vi "Final_DAQ_v2.vi"() -> ()   [LabVIEW 2019]
uses:
  src/class/mqtt/mqttTypedef/mqttBroker.ctl
  src/class/mqtt/mqttTypedef/mqttConnectionFlags.ctl
  src/class/mqtt/mqttTypedef/mqttWillInformation.ctl
  src/class/mqtt/mqttConfigFunction.ctl
  src/class/mqtt/mqttTXqueue/mqttTXdataQueueFunction.ctl
  src/class/mqtt/mqttTXqueue/mqttRXsubscriptionEventFunction.ctl
  src/class/mqtt/mqtt.lvclass
panel:
  out "電暖爐":bool
  out "電扇":bool
  out "電燈":bool
  out "開門 Flag":bool
  out "電暖爐-M":bool
  out "電扇-M":bool
  out "開門":bool
  out "電燈-M":bool
  out "溫度過低":bool
  out "溫度過高":bool
  out "Boolean":bool
  out "old-temp":dbl
  out "Numeric 2":dbl
  out "subscripts-status":bool
  out "Publish Topic":string
  out "Publish Data":string
  out "溫度上限(*C)":dbl
  out "溫度下限(*C)":dbl
  out "Subscripts Topic":string
  out "Subscripts Data":string
  out "F-format string":string
  out "now-temp":dbl
  out "Thermometer":dbl(slide) scale=0.0..40.0
  in  "stop":bool
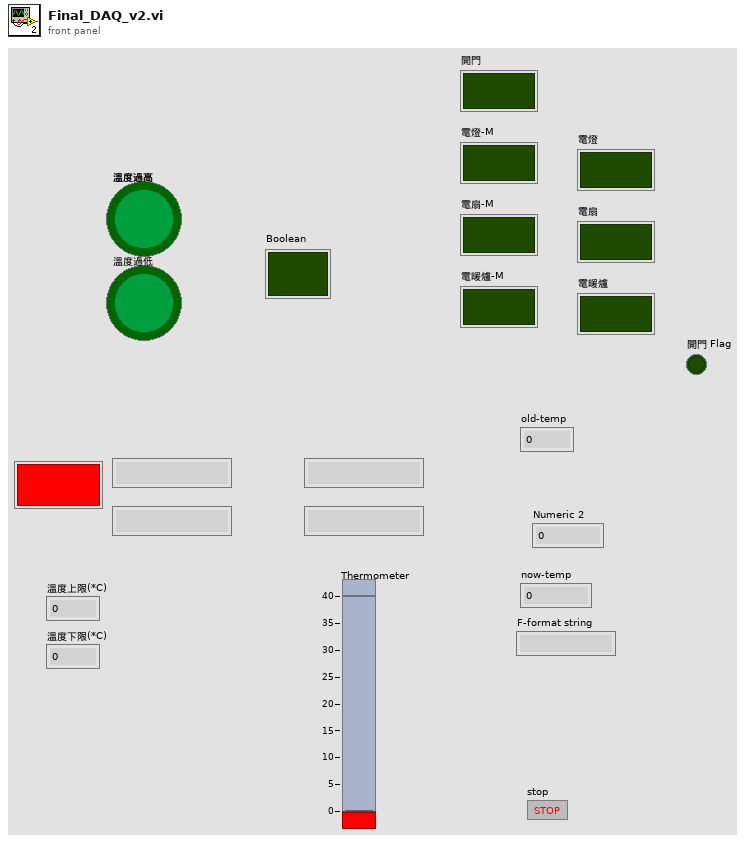
[diagram p1: front panel]
types:
  T1 = typedef "mqttRXsubscriptionEventFunction.ctl" = enum16{"init", "deinit", "getEventRef", "event"}
  T2 = typedef "mqttTXdataQueueFunction.ctl" = enum16{"init", "deinit", "getQueue", "enqueue"}
  T3 = typedef "mqtt.lvclass/mqttConfigFunction.ctl" = enum16{"init", "deinit", "set", "get"}
  T4 = typedef "mqttWillInformation.ctl" = cluster{"User Name":string, "Password":string}
  T5 = typedef "mqttConnectionFlags.ctl" = cluster{"reserved":bool, "clean session":bool, "will flag":bool, "willQOS":enum8{"At most once", "At least once", "Exactly once", "Reserved"}, "will retain":bool, "password":bool, "user name":bool}
  T6 = typedef "mqttBroker.ctl" = cluster{"address":string, "port":u16, "connTimeout":i32, "writeTimeout":i32, "readTimeout":i32, "subTimeout":i32}
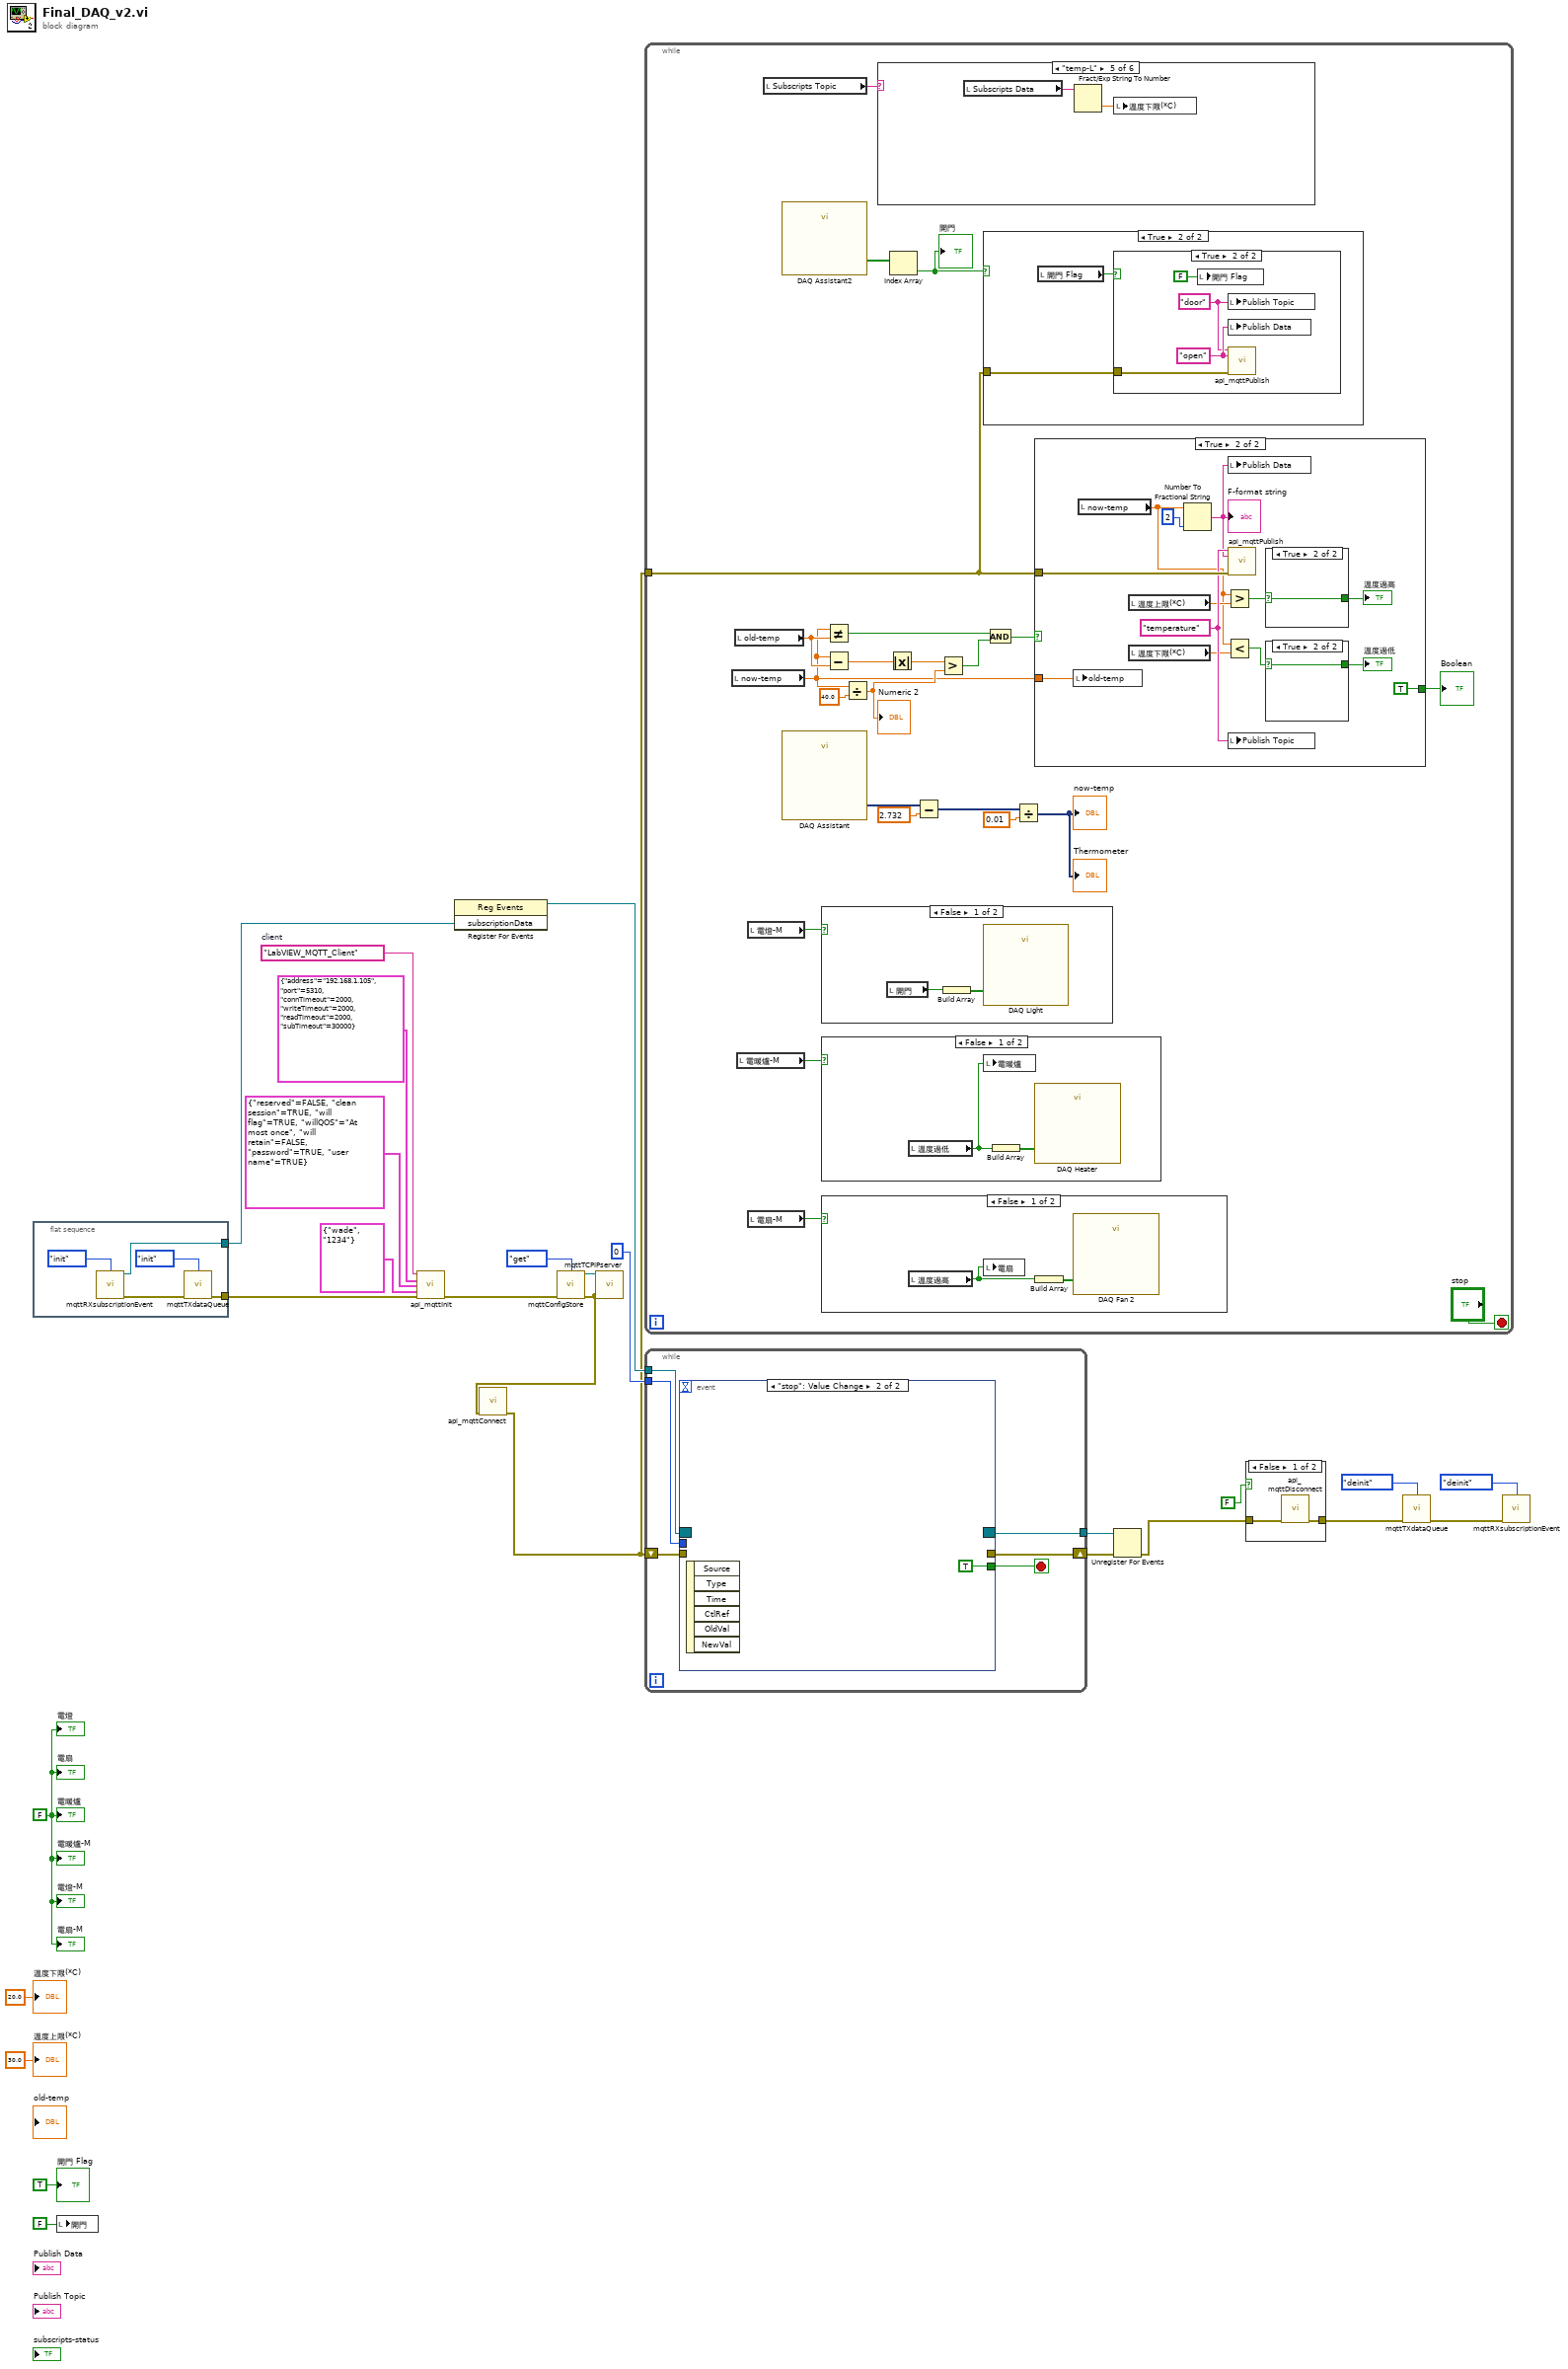
[diagram p0: block diagram]
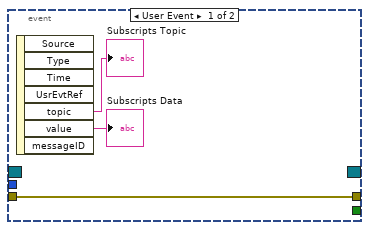
[diagram p3: hidden frame]
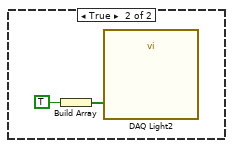
[diagram p4: hidden frame]
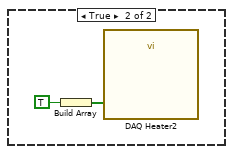
[diagram p5: hidden frame]
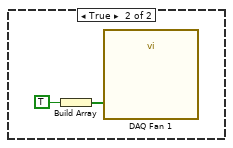
[diagram p6: hidden frame]
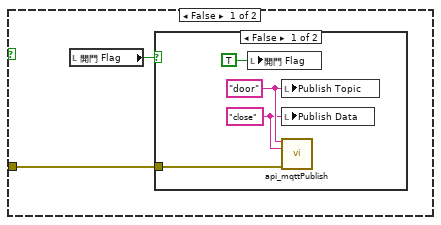
[diagram p7: hidden frame]
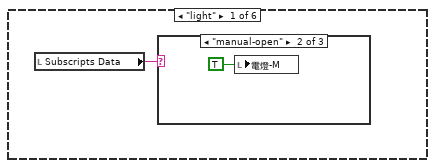
[diagram p10: hidden frame]
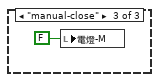
[diagram p12: hidden frame]
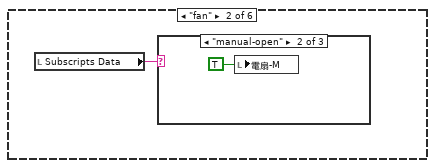
[diagram p13: hidden frame]
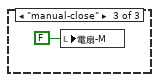
[diagram p15: hidden frame]
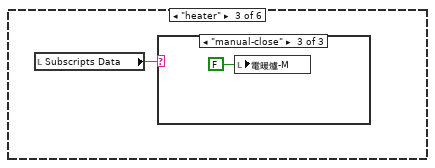
[diagram p16: hidden frame]
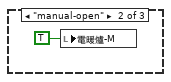
[diagram p18: hidden frame]
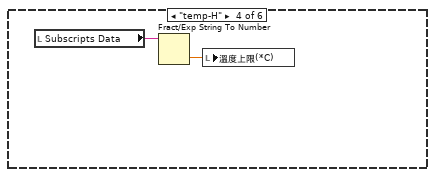
[diagram p19: hidden frame]
diagram:
  w16 = "LabVIEW_MQTT_Client"  # client
  w19 = FALSE
  n1 = flat-sequence {
    tunnel: [w30] -> w11
    tunnel: [w27] -> w26
    frame #0 {
      n2 = call "mqttRXsubscriptionEvent.vi"("function"=mqttRXsubscriptionEventFunction."init") -> ("subscriptionData"=w27:refnum<user-event>, "error out"=w29:errorcluster)  [unwired: 13 in]
      n3 = call "mqttTXdataQueue.vi"("function"=mqttTXdataQueueFunction."init", "error in (no error)"=w29) -> ("error out"=w30:errorcluster)  [unwired: 12 in, 1 out]
    }
  }
  n4 = local write "開門"(FALSE ("開門")) -> ()
  n5 = call "api_mqttInit.vi"("client"=w16, "broker"=T6 {"address"="192.168.1.105", "port"=5310, "connTimeout"=2000, "writeTimeout"=2000, "readTimeout"=2000, "subTimeout"=30000}, "connFlags"=T5 {"reserved"=FALSE, "clean session"=TRUE, "will flag"=TRUE, "willQOS"=enum."At most once", "will retain"=FALSE, "password"=TRUE, "user name"=TRUE}, "User Info"=T4 {"User Name"="wade", "Password"="1234"}, "error in (no error)"=w11) -> ("error out"=w17:errorcluster)  [unwired: 10 in]
  n6 = register-events(w26) -> (reference out=w25:refnum<event-registration>)  [unwired: 2 in, 1 out]
  n7 = call "mqttConfigStore.vi"("function"=mqttConfigFunction."get", "error in (no error)"=w17) -> ("mqtt.lvclass out"=w12:refnum<class "mqtt.lvclass">, "error out"=w4:errorcluster)  [unwired: 12 in]
  n8 = call "api_mqttConnect.vi"("error in (no error)"=w4) -> ("error out"=w3:errorcluster)  [unwired: 11 in, 3 out]
  n9 = call "mqttTCPIPserver.vi"("mqtt.lvclass"=w12, "error in (no error)"=w4) -> ()  [unwired: 12 in, 2 out]
  n10 = while {
    tunnel: w3 -> [w37]
    stop <- "stop" stop-if-true
    n11 = local read "now-temp"() -> (w41:dbl)
    n12 = local read "old-temp"() -> (w47:dbl)
    n13 = local read "電暖爐-M"() -> (w34:bool)
    n14 = local read "電燈-M"() -> (w33:bool)
    n15 = local read "電扇-M"() -> (w35:bool)
    n16 = local read "Subscripts Topic"() -> (w38:string)
    n17 = call "DAQ Assistant2"() -> ("data"=w49:bool[])  [unwired: 17 in, 2 out]
    n18 = call "DAQ Assistant"() -> ("data"=w50:dynamicdata)  [unwired: 17 in, 2 out]
    n19 = case shown="False" w33 {
      frame False {
        n20 = local read "開門"() -> (w56:bool)
        n21 = Build Array(w56) -> (w55:bool[])
        n22 = call "DAQ Light"("data"=w55) -> ()  [unwired: 17 in, 2 out]
      }
      frame True {
        n23 = Build Array(TRUE) -> (w57:bool[])
        n24 = call "DAQ Light2"("data"=w57) -> ()  [unwired: 17 in, 2 out]
      }
    }
    n25 = case shown="False" w34 {
      frame False {
        n26 = local read "溫度過低"() -> (w60:bool)
        n27 = local write "電暖爐"(w60) -> ()
        n28 = Build Array(w60) -> (w59:bool[])
        n29 = call "DAQ Heater"("data"=w59) -> ()  [unwired: 17 in, 2 out]
      }
      frame True {
        n30 = Build Array(TRUE) -> (w61:bool[])
        n31 = call "DAQ Heater2"("data"=w61) -> ()  [unwired: 17 in, 2 out]
      }
    }
    n32 = case shown="False" w35 {
      frame False {
        n33 = local read "溫度過高"() -> (w63:bool)
        n34 = local write "電扇"(w63) -> ()
        n35 = Build Array(w63) -> (w64:bool[])
        n36 = call "DAQ Fan 2"("data"=w64) -> ()  [unwired: 17 in, 2 out]
      }
      frame True {
        n37 = Build Array(TRUE) -> (w66:bool[])
        n38 = call "DAQ Fan 1"("data"=w66) -> ()  [unwired: 17 in, 2 out]
      }
    }
    n39 = Not Equal?(x=w41, y=w47) -> (x != y?=w48:bool)
    n40 = Subtract(x=w41, y=w47) -> (x-y=w46:dbl)
    n41 = Divide(x=w41, y=40.0) -> (x/y=w44:dbl)
    "Numeric 2" <- w44
    n42 = case shown="\"temp-L\"" w38 {
      frame "light" {
        n43 = local read "Subscripts Data"() -> (w79:string)
        n44 = case shown="\"manual-open\"" w79 {
          frame "None", Default {
          }
          frame "manual-open" {
            n45 = local write "電燈-M"(TRUE ("電燈")) -> ()
          }
          frame "manual-close" {
            n46 = local write "電燈-M"(FALSE ("電燈")) -> ()
          }
        }
      }
      frame "fan" {
        n47 = local read "Subscripts Data"() -> (w82:string)
        n48 = case shown="\"manual-open\"" w82 {
          frame "None", Default {
          }
          frame "manual-open" {
            n49 = local write "電扇-M"(TRUE ("電扇")) -> ()
          }
          frame "manual-close" {
            n50 = local write "電扇-M"(FALSE ("電扇")) -> ()
          }
        }
      }
      frame "heater" {
        n51 = local read "Subscripts Data"() -> (w85:string)
        n52 = case shown="\"manual-close\"" w85 {
          frame "None", Default {
          }
          frame "manual-open" {
            n53 = local write "電暖爐-M"(TRUE ("電暖爐")) -> ()
          }
          frame "manual-close" {
            n54 = local write "電暖爐-M"(FALSE ("電暖爐")) -> ()
          }
        }
      }
      frame "temp-H" {
        n55 = local read "Subscripts Data"() -> (w89:string)
        n56 = Fract/Exp String To Number(string=w89) -> (number=w88:dbl)  [unwired: 3 in, 1 out]
        n57 = local write "溫度上限(*C)"(w88) -> ()
      }
      frame "temp-L" {
        n58 = local read "Subscripts Data"() -> (w91:string)
        n59 = Fract/Exp String To Number(string=w91) -> (number=w90:dbl)  [unwired: 3 in, 1 out]
        n60 = local write "溫度下限(*C)"(w90) -> ()
      }
      frame "none", Default {
      }
    }
    n61 = Absolute Value(x=w46) -> (abs(x)=w45:dbl)
    n62 = Index Array(array=w49) -> (element=w36:bool)  [unwired: 1 in]
    "開門" <- w36
    n63 = Subtract(x=w50, y=2.732) -> (x-y=w52:dynamicdata)
    n64 = Greater?(x=w45, y=w44) -> (0:w43:bool)
    n65 = case shown="True" w36 {
      tunnel: w37 -> [w67 w74]
      frame False {
        n66 = local read "開門 Flag"() -> (w68:bool)
        n67 = case shown="False" w68 {
          tunnel: w67 -> [w69 _]
          frame False {
            w70 = "close"
            w71 = "door"
            n68 = local write "開門 Flag"(TRUE ("開門 Flag")) -> ()
            n69 = local write "Publish Topic"(w71) -> ()
            n70 = local write "Publish Data"(w70) -> ()
            n71 = call "api_mqttPublish.vi"("topic"=w71, "value"=w70, "error in (no error)"=w69) -> ()  [unwired: 11 in, 2 out]
          }
          frame True {
          }
        }
      }
      frame True {
        n72 = local read "開門 Flag"() -> (w73:bool)
        n73 = case shown="True" w73 {
          tunnel: w74 -> [_ w76]
          frame False {
          }
          frame True {
            w78 = "open" ("value")
            w77 = "door" ("topic")
            n74 = local write "開門 Flag"(FALSE ("開門 Flag")) -> ()
            n75 = local write "Publish Topic"(w77) -> ()
            n76 = local write "Publish Data"(w78) -> ()
            n77 = call "api_mqttPublish.vi"("topic"=w77, "value"=w78, "error in (no error)"=w76) -> ()  [unwired: 11 in, 2 out]
          }
        }
      }
    }
    n78 = And(x=w48, y=w43) -> (x .and. y?=w42:bool)
    n79 = Divide(x=w52, y=0.01) -> (x/y=→"Thermometer" →"now-temp":dynamicdata)
    n80 = case shown="True" w42 {
      tunnel: w41 -> [_ w105]
      tunnel: [FALSE ("Boolean") TRUE ("Boolean")] -> w40
      tunnel: w37 -> [_ w103]
      frame False {
      }
      frame True {
        w101 = "temperature" ("topic")
        n81 = local write "old-temp"(w105) -> ()
        n82 = local read "now-temp"() -> (w95:dbl)
        n83 = local read "溫度上限(*C)"() -> (w99:dbl)
        n84 = local read "溫度下限(*C)"() -> (w96:dbl)
        n85 = Number To Fractional String(number=w95, precision (6)=i16 2) -> (F-format string=w100:string)  [unwired: 2 in]
        "F-format string" <- w100
        n86 = Greater?(x=w95, y=w99) -> (0:w98:bool)
        n87 = Less?(x=w95, y=w96) -> (x < y?=w97:bool)
        n88 = local write "Publish Data"(w100) -> ()
        n89 = call "api_mqttPublish.vi"("topic"=w101, "value"=w100, "error in (no error)"=w103) -> ()  [unwired: 11 in, 2 out]
        n90 = local write "Publish Topic"(w101) -> ()
        n91 = case shown="True" w98 {
          selector: w98 -> [w108 w109]
          tunnel: [w108 w109] -> w94
          frame False {
          }
          frame True {
          }
        }
        "溫度過高" <- w94
        n92 = case shown="True" w97 {
          selector: w97 -> [w106 w107]
          tunnel: [w106 w107] -> w93
          frame False {
          }
          frame True {
          }
        }
        "溫度過低" <- w93
      }
    }
    "Boolean" <- w40
  }
  n93 = while {
    tunnel: w25 -> [w112]
    shift-right: [w113] -> w24
    shift-left: w3 -> [w114]
    tunnel: [w111] -> w23
    tunnel: 0 -> [w110]
    stop <- w115 stop-if-true
    n94 = event shown="[1] \"stop\": Value Change" {
      selector: w112 -> [_ _]
      dyn-events: [_ _] -> w111
      timeout: _ -> [_ _]
      tunnel: [_ TRUE] -> w115
      tunnel: w114 -> [w116 _]
      tunnel: [w116 _] -> w113
      tunnel: w110 -> [_ _]
      event User Event {
        n95 = event-data() -> ("topic"=→"Subscripts Topic":string, "value"=→"Subscripts Data":string)  [unwired: 1 in, 5 out]
      }
      event "stop": Value Change {
        n96 = event-data() -> ()  [unwired: 1 in, 6 out]
      }
    }
  }
  n97 = Unregister For Events(event registration refnum=w23, error in=w24) -> (error out=w6:errorcluster)
  n98 = case shown="False" FALSE {
    tunnel: [w121 w122] -> w9
    tunnel: w6 -> [w120 w122]
    frame False {
      n99 = call "api_mqttDisconnect.vi"("error in (no error)"=w120) -> ("error out"=w121:errorcluster)  [unwired: 13 in, 1 out]
    }
    frame True {
    }
  }
  n100 = call "mqttTXdataQueue.vi"("function"=mqttTXdataQueueFunction."deinit", "error in (no error)"=w9) -> ("error out"=w7:errorcluster)  [unwired: 12 in, 1 out]
  n101 = call "mqttRXsubscriptionEvent.vi"("function"=mqttRXsubscriptionEventFunction."deinit", "error in (no error)"=w7) -> ()  [unwired: 12 in, 2 out]
  "電扇-M" <- w19
  "電暖爐-M" <- w19
  "電燈-M" <- w19
  "開門 Flag" <- TRUE ("開門 Flag")
  "電燈" <- w19
  "電扇" <- w19
  "電暖爐" <- w19
  "溫度上限(*C)" <- 30.0 ("溫度上限(*C)")
  "溫度下限(*C)" <- 20.0 ("溫度下限(*C)")
